vi "BRig_RT__Case_Exp__State_ENLPre__v4.vi"(4 "input_arrTrig":bool[](array[boolean]), 6 "input_ENL2":bool, 7 "input_I_lick":bool, 8 "input_dataExp":u16[](array[numeric]), 9 "input_dataTrial":u16[][](array[numeric]), 11 "input_dataCurrent":u16[](array[numeric])) -> (0 "output_arrTrig":bool[](array[boolean]), 1 "output_dataTrial":u16[][](array[numeric]), 3 "output_dataCurrent":u16[](array[numeric]), 5 "output_state":T1)   [LabVIEW 2014]
uses:
  myRIO_BRig_RT__Case_Exp_stateList.ctl
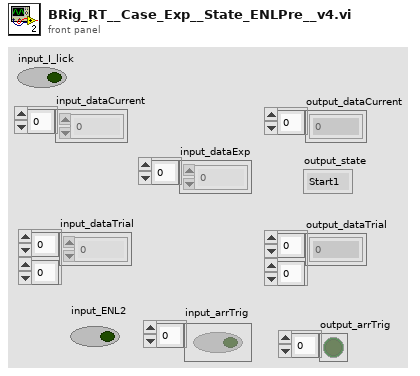
[diagram p1: front panel]
types:
  T1 = typedef "myRIO_BRig_RT__Case_Exp_stateList.ctl" = enum16{"Start1", "Start2", "Start3", "saveSettings1", "saveSettings2", "saveSettings3", "saveSettings4", "saveSettings_LC_ENL_l1", "saveSettings_LC_ENL_l2", "saveSettings_LC_Cue_l1", "saveSettings_LC_Cue_l2", "saveSettings6_LC_l1_Other", "SaveSettings6_LC_l2_Other", "setSettings_Audio", "setSettings_Laser", "initBlock_pre", "initBlock", "initBlock2", "initBlock_post", "initTrial_pre", "initTrial", "initTrial2", "initTrial3", "initTrial4", "initTrial_LC_ENL1", "initTrial_LC_Cue1", "initTrial_LC_Cue1_2", "initTrial_LC_Sel", "initTrial_post", "ENL1_pre", "ENL1", "ENL1_post", "ENL1Penalty_pre", "ENL1Penalty", "ENL2_pre", "ENL2", "ENL2Penalty_pre", "ENL2Penalty", "Cue1_pre", "Cue1", "Cue1_post", "Cue1Penalty_pre", "Cue1Penalty", "Cue2_pre", "Cue2", "Cue2Penalty_pre", "Cue2Penalty", "Selection_pre", "Selection", "Select_post", "SelectReward_pre", "SelectReward", "SelectRewardPost_pre", "SelectRewardPost", "SelectWrong_pre", "SelectWrong", "SelectWrong_post", "SelectTimeout_pre", "SelectTimeout", "SelectTimeout_post", "endTrial_pre", "endTrial1", "endTrial2", "endTrial3", "endTrial_post", "endBlock_pre", "endBlock", "endBlock_post", "endExp", "commConnect", "commUpload_pre", "commUpload_dataBlock", "commUpload_dataCurrent", "commUpload_dataExp", "commUpload_dataLC", "commUpload_dataTrial", "commUpload_post", "saveData_pre", "saveData_dataBlock", "saveData_dataCurrent", "saveData_dataExp", "saveData_dataLC", "saveData_dataTrial", "saveData_post", "empty_endBlock1", "empty_endBlock2", "empty_endTrial1", "empty_endTrial2", "empty_endTrial3", "empty_endTrial4", "empty_endTrial5", "dummyState", "dummyState_endBlock", "FreeReward_pre", "FreeReward", "FreeRewardPost_pre", "FreeRewardPost"}
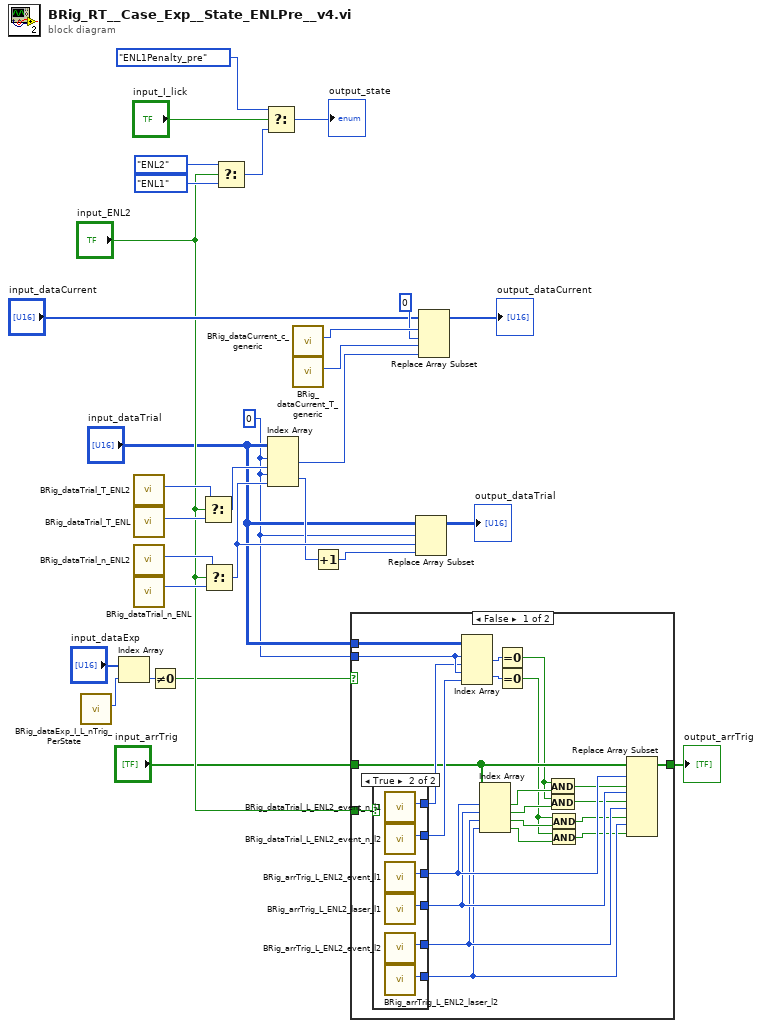
[diagram p0: block diagram]
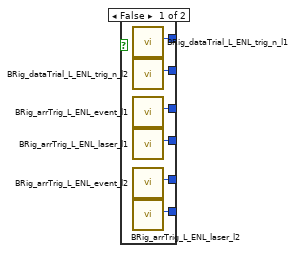
[diagram p2: hidden frame]
diagram:
  w2 = 0
  n1 = call "BRig_dataExp_I_L_nTrig_PerState.vi"() -> ("output_I_L_nTrig_PerState"=w9:i32)  [unwired: 11 in]
  n2 = Index Array(array="input_dataExp", index=w9) -> (element=w8:u16)
  n3 = call "BRig_dataTrial_T_ENL2.vi"() -> ("output_T_ENL2"=w11:i32)  [unwired: 11 in]
  n4 = call "BRig_dataTrial_T_ENL.vi"() -> ("output_T_ENL"=w13:i32)  [unwired: 11 in]
  n5 = call "BRig_dataTrial_n_ENL2.vi"() -> ("output_ENL2_n"=w16:i32)  [unwired: 11 in]
  n6 = call "BRig_dataTrial_n_ENL.vi"() -> ("output_ENL_n"=w15:i32)  [unwired: 11 in]
  n7 = Not Equal To 0?(x=w8) -> (x != 0?=w4:bool)
  n8 = Select(t=w11, s="input_ENL2", f=w13) -> (s? t:f=w12:i32)
  n9 = Select(t=w16, s="input_ENL2", f=w15) -> (s? t:f=w14:i32)
  n10 = Select(t=myRIO_BRig_RT__Case_Exp_stateList."ENL2" ("Enum"), s="input_ENL2", f=myRIO_BRig_RT__Case_Exp_stateList."ENL1" ("Enum")) -> (s? t:f=w17:T1)
  n11 = Select(t=myRIO_BRig_RT__Case_Exp_stateList."ENL1Penalty_pre" ("Enum"), s="input_I_lick", f=w17) -> (s? t:f=→"output_state":T1)
  n12 = Index Array(array="input_dataTrial", index (row) #1=w2, index (col) #1=w12, index (row) #2=w2, index (col) #2=w14) -> (element #1=w28:u16, element #2=w7:u16)
  n13 = call "BRig_dataCurrent_c_generic.vi"() -> ("output_count_generic"=w30:i32)  [unwired: 11 in]
  n14 = call "BRig_dataCurrent_T_generic.vi"() -> ("output_T_generic"=w29:i32)  [unwired: 11 in]
  n15 = Increment(x=w7) -> (x+1=w22:u16)
  n16 = case shown="False" w4 {
    tunnel: "input_ENL2" -> [w53 _]
    tunnel: "input_arrTrig" -> [w46 w66]
    tunnel: [w45 w66] -> w1
    tunnel: "input_dataTrial" -> [w52 _]
    tunnel: w2 -> [w51 _]
    frame False {
      n17 = case shown="True" w53 {
        tunnel: [w59 w65] -> w38
        tunnel: [w58 w64] -> w37
        tunnel: [w57 w63] -> w36
        tunnel: [w56 w62] -> w35
        tunnel: [w55 w61] -> w50
        tunnel: [w54 w60] -> w49
        frame False {
          n18 = call "BRig_dataTrial_L_ENL_trig_n_l1.vi"() -> ("output_L_ENL_trig_n_l1"=w55:i32)  [unwired: 11 in]
          n19 = call "BRig_dataTrial_L_ENL_trig_n_l2.vi"() -> ("output_L_ENL_trig_n_l2"=w54:i32)  [unwired: 11 in]
          n20 = call "BRig_arrTrig_L_ENL_event_l1.vi"() -> ("output_L_ENL_event_l1"=w59:i32)  [unwired: 11 in]
          n21 = call "BRig_arrTrig_L_ENL_laser_l1.vi"() -> ("output_L_ENL_laserTrig_l1"=w58:i32)  [unwired: 11 in]
          n22 = call "BRig_arrTrig_L_ENL_event_l2.vi"() -> ("output_L_ENL_event_l2"=w57:i32)  [unwired: 11 in]
          n23 = call "BRig_arrTrig_L_ENL_laser_l2.vi"() -> ("output_L_ENL_laserTrig_l2"=w56:i32)  [unwired: 11 in]
        }
        frame True {
          n24 = call "BRig_dataTrial_L_ENL2_event_n_l1.vi"() -> ("output_L_ENL2_event_n_l1"=w61:i32)  [unwired: 11 in]
          n25 = call "BRig_dataTrial_L_ENL2_event_n_l2.vi"() -> ("output_L_ENL2_event_n_l2"=w60:i32)  [unwired: 11 in]
          n26 = call "BRig_arrTrig_L_ENL2_event_l1.vi"() -> ("output_L_ENL2_event_l1"=w65:i32)  [unwired: 11 in]
          n27 = call "BRig_arrTrig_L_ENL2_laser_l1.vi"() -> ("output_L_ENL2_laserTrig_l1"=w64:i32)  [unwired: 11 in]
          n28 = call "BRig_arrTrig_L_ENL2_event_l2.vi"() -> ("output_L_ENL2_event_l2"=w63:i32)  [unwired: 11 in]
          n29 = call "BRig_arrTrig_L_ENL2_laser_l2.vi"() -> ("output_L_ENL2_laserTrig_l2"=w62:i32)  [unwired: 11 in]
        }
      }
      n30 = Index Array(array=w52, index (row) #1=w51, index (col) #1=w50, index (row) #2=w51, index (col) #2=w49) -> (element #1=w48:u16, element #2=w47:u16)
      n31 = Index Array(array=w46, index #1=w38, index #2=w37, index #3=w36, index #4=w35) -> (element #1=w44:bool, element #2=w43:bool, element #3=w41:bool, element #4=w40:bool)
      n32 = Equal To 0?(x=w48) -> (x = 0?=w42:bool)
      n33 = Equal To 0?(x=w47) -> (x = 0?=w39:bool)
      n34 = And(x=w42, y=w44) -> (x .and. y?=w34:bool)
      n35 = And(x=w42, y=w43) -> (x .and. y?=w33:bool)
      n36 = And(x=w39, y=w41) -> (x .and. y?=w32:bool)
      n37 = And(x=w39, y=w40) -> (x .and. y?=w31:bool)
      n38 = Replace Array Subset(array=w46, new element #1=w34, index #1=w38, new element #2=w33, index #2=w37, new element #3=w32, index #3=w36, new element #4=w31, index #4=w35) -> (w45:bool[])
    }
    frame True {
    }
  }
  "output_arrTrig" <- w1
  n39 = Replace Array Subset(array="input_dataTrial", new element=w22, index (row)=w2, index (col)=w14) -> (→"output_dataTrial":u16[][])
  n40 = Replace Array Subset(array="input_dataCurrent", new element #1=u16 0 ("new element/subarray"), index #1=w30, new element #2=w28, index #2=w29) -> (→"output_dataCurrent":u16[])
